vi "Configure Waveform Modulation (FSK).vi"(6 "FSK Rate (1000 Hz)":dbl=1000.0, 8 "error in (no error)":errorcluster, 9 "Hop Frequency (2000 Hz)":dbl=2000.0, 10 "Waveform Generator Number (1: Waveform Generator 1)":i32(ring)=1 items=["Waveform Generator 1"=1], 11 "VISA resource name":refnum<visa-resource-name>) -> (0 "error out":errorcluster, 3 "VISA resource name out":refnum<visa-resource-name>)   [LabVIEW 2017, in "Agilent 2000 3000 X-Series.lvlib"]
doc: "Configures the waveform modulation FSK."
uses:
  Agilent 2000 3000 X-Series.lvlib
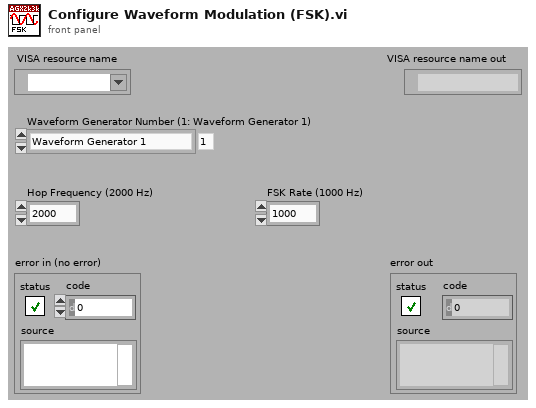
[diagram p1: front panel]
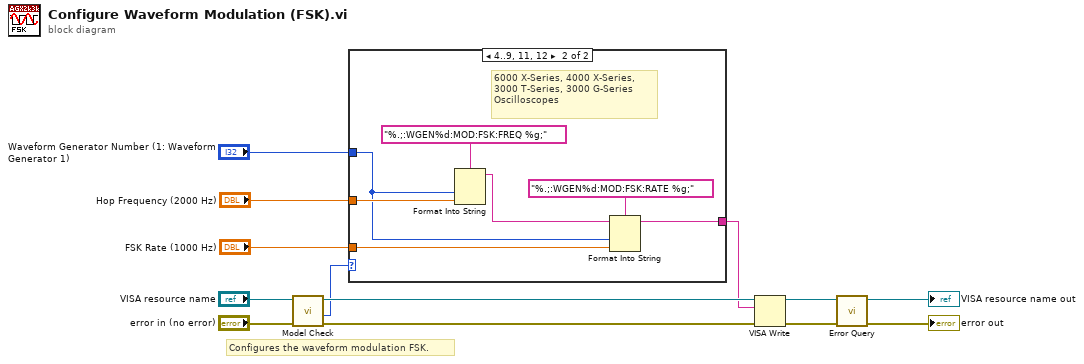
[diagram p0: block diagram]
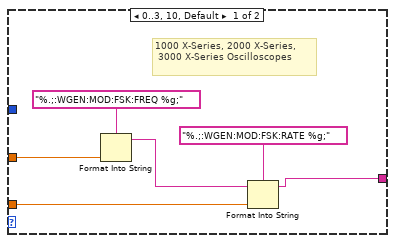
[diagram p2: hidden frame]
diagram:
  # "Configures the waveform modulation FSK."
  n1 = call "Model Check.vi"("error in (no error)"="error in (no error)", "VISA resource name"="VISA resource name") -> ("error out"=w3:errorcluster, "Model"=w2:i32, "VISA resource name out"=w4:refnum<visa-resource-name>)  [unwired: 7 out]
  n2 = case shown="4..9, 11, 12" w2 {
    tunnel: "Hop Frequency (2000 Hz)" -> [w17 w23]
    tunnel: "FSK Rate (1000 Hz)" -> [w18 w24]
    tunnel: "Waveform Generator Number (1: Waveform Generator 1)" -> [_ w22]
    tunnel: [w14 w20] -> w1
    frame 0..3, 10, Default {
      # "1000 X-Series, 2000 X-Series,\n 3000 X-Series Oscilloscopes"
      n3 = Format Into String(format string="%.;:WGEN:MOD:FSK:FREQ %g;", w17) -> (resulting string=w16:string)  [unwired: 2 in, 1 out]
      n4 = Format Into String(format string="%.;:WGEN:MOD:FSK:RATE %g;", initial string=w16, w18) -> (resulting string=w14:string)  [unwired: 1 in, 1 out]
    }
    frame 4..9, 11, 12 {
      # "6000 X-Series, 4000 X-Series, 3000 T-Series, 3000 G-Series Oscilloscopes"
      n5 = Format Into String(format string="%.;:WGEN%d:MOD:FSK:FREQ %g;", w22, w23) -> (resulting string=w21:string)  [unwired: 2 in, 1 out]
      n6 = Format Into String(format string="%.;:WGEN%d:MOD:FSK:RATE %g;", initial string=w21, w22, w24) -> (resulting string=w20:string)  [unwired: 1 in, 1 out]
    }
  }
  n7 = VISA Write(VISA resource name=w4, write buffer=w1, error in (no error)=w3) -> (VISA resource name out=w10:refnum<visa-resource-name>, error out=w9:errorcluster)  [unwired: 1 out]
  n8 = call "Error Query.vi"("error in (no error)"=w9, "VISA resource name"=w10) -> ("error out"=→"error out":errorcluster, "VISA resource name out"=→"VISA resource name out":refnum<visa-resource-name>)  [unwired: 6 in, 2 out]
